vi "CreatePrivateEvents.vi"(8 "error in (no error)":errorcluster, 11 "RemoteControl":refnum<class "RemoteControl.lvclass">) -> (0 "error out":errorcluster, 3 "RemoteControl out":refnum<class "RemoteControl.lvclass">)   [LabVIEW 2016, in "RemoteControl.lvclass"]
doc: "---------------------------------------------------------------\nJKI State Machine Objects™\nhttp://jki.net/state-machine-objects/\nCopyright (C) 2005-2015, JKI <info@jki.net>\nALL RIGHTS RESERVEDJKI State Machine Objects (SMO) 1.0.0.4\nJKI - JKI\nCopyright (c) 2015, JKI"
uses:
  RemoteControl.lvclass
  Typedefs/PrivateEvents--RemoteControl.setAllowedRemoteAddress.ctl
  Typedefs/PrivateEvents--RemoteControl.setAO.ctl
  Typedefs/PrivateEvents--RemoteControl.setAI.ctl
  Typedefs/PrivateEvents--RemoteControl.setResults.ctl
  Typedefs/PrivateEvents--RemoteControl.setTrigger.ctl
  Typedefs/PrivateEvents--RemoteControl.setAOconfig.ctl
  Typedefs/AO-cluster.ctl
  Typedefs/AO_Amp-array.ctl
  Typedefs/AO_DC-array.ctl
  Typedefs/AO_f-array.ctl
  Typedefs/AO_phi-array.ctl
  Typedefs/Function-array.ctl
  Typedefs/Function-enum.ctl
  Typedefs/PrivateEvents--RemoteControl.setREFconfig.ctl
  Typedefs/REF-cluster.ctl
  Typedefs/REF_f-array.ctl
  Typedefs/REF_phi-array.ctl
  Typedefs/PrivateEvents--RemoteControl.setReset.ctl
  Typedefs/PrivateEvents--RemoteControl.setIVmode.ctl
  RemoteControl.lvclass/RemoteControl.ctl
  <vilib>/JKI/JKI SMO/SMO/SMO.lvclass
panel:
  # "For instructions on how to use the JKI State Machine Objects, examples and video tutorials, visit:\nhttp://jki.net/state-machine-objects/\n\nJKI State Machine Objects™\nhttp://jki.net/state-machine-objects/\nCopyright (C) 2005-2015, JKI <info@jki.net>\nALL RIGHTS RESERVED"
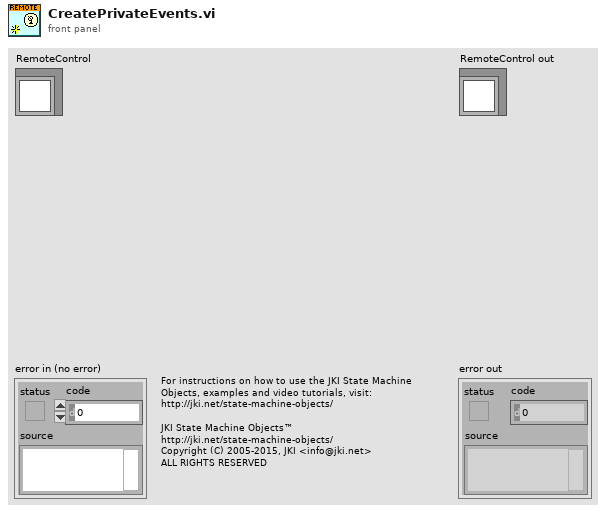
[diagram p1: front panel]
types:
  T1 = typedef "RemoteControl.lvclass/PrivateEvents--RemoteControl.setIVmode.ctl" = bool
  T2 = typedef "RemoteControl.lvclass/PrivateEvents--RemoteControl.setReset.ctl" = bool
  T3 = typedef "RemoteControl.lvclass/PrivateEvents--RemoteControl.setREFconfig.ctl" = cluster{"Channels: Lockin":T4}
  T4 = typedef "REF-cluster.ctl" = cluster{"REF f (Hz)":T5, "REF phi (deg)":T6}
  T5 = typedef "REF_f-array.ctl" = dbl[]
  T6 = typedef "REF_phi-array.ctl" = dbl[]
  T7 = typedef "RemoteControl.lvclass/PrivateEvents--RemoteControl.setAOconfig.ctl" = cluster{"Channels: AO":T8}
  T8 = typedef "AO-cluster.ctl" = cluster{"AO amp (V)":T9, "AO DC (V)":T10, "AO f (Hz)":T11, "AO phi (deg)":T12, "function":T13}
  T9 = typedef "AO_Amp-array.ctl" = dbl[]
  T10 = typedef "AO_DC-array.ctl" = dbl[]
  T11 = typedef "AO_f-array.ctl" = dbl[]
  T12 = typedef "AO_phi-array.ctl" = dbl[]
  T13 = typedef "Function-array.ctl" = T14[]
  T14 = typedef "Function-enum.ctl" = enum16{"Sine Wave", "Triangle Wave", "Square Wave", "Sawtooth Wave"}
  T15 = typedef "RemoteControl.lvclass/PrivateEvents--RemoteControl.setTrigger.ctl" = bool
  T16 = typedef "RemoteControl.lvclass/PrivateEvents--RemoteControl.setResults.ctl" = dbl[][]
  T17 = typedef "RemoteControl.lvclass/PrivateEvents--RemoteControl.setAI.ctl" = waveform(dbl)[]
  T18 = typedef "RemoteControl.lvclass/PrivateEvents--RemoteControl.setAO.ctl" = waveform(dbl)[]
  T19 = typedef "RemoteControl.lvclass/PrivateEvents--RemoteControl.setAllowedRemoteAddress.ctl" = string
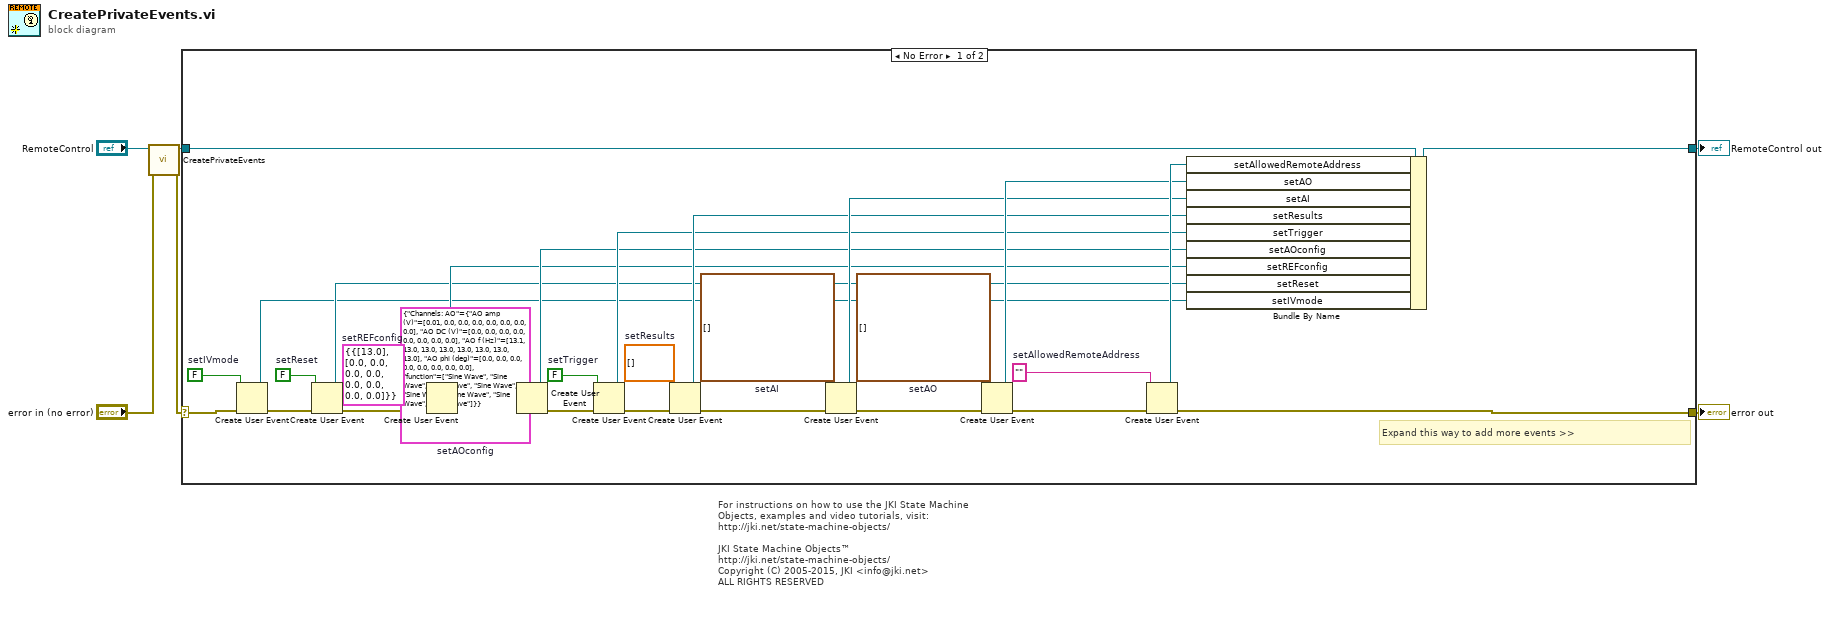
[diagram p0: block diagram]
diagram:
  # "For instructions on how to use the JKI State Machine Objects, examples and video tutorials, visit:\nhttp://jki.net/state-machine-objects/\n\nJKI State Machine Objects™\nhttp://jki.net/state-machine-objects/\nCopyright (C) 2005-2015, JKI <info@jki.net>\nALL RIGHTS RESERVED"
  n1 = call-parent "CreatePrivateEvents.vi"("error in (no error)"="error in (no error)", "SMO"="RemoteControl") -> ("error out"=w1:errorcluster, "SMO out"=w3:refnum<class "RemoteControl.lvclass">)  [unwired: 8 in]
  n2 = case shown="No Error" w1 {
    selector: w1 -> [w35 w38]
    tunnel: [w33 w38] -> w5
    tunnel: [w34 w37] -> w6
    tunnel: w3 -> [w36 w37]
    frame No Error {
      w8 = T1 FALSE  # setIVmode
      w11 = T2 FALSE  # setReset
      w14 = T3 {"Channels: Lockin"={"REF f (Hz)"=[13.0], "REF phi (deg)"=[0.0, 0.0, 0.0, 0.0, 0.0, 0.0, 0.0, 0.0]}}  # setREFconfig
      w17 = T7 {"Channels: AO"={"AO amp (V)"=[0.01, 0.0, 0.0, 0.0, 0.0, 0.0, 0.0, 0.0], "AO DC (V)"=[0.0, 0.0, 0.0, 0.0, 0.0, 0.0, 0.0, 0.0], "AO f (Hz)"=[13.1, 13.0, 13.0, 13.0, 13.0, 13.0, 13.0, 13.0], "AO phi (deg)"=[0.0, 0.0, 0.0, 0.0, 0.0, 0.0, 0.0, 0.0], "function"=[enum."Sine Wave", enum."Sine Wave", enum."Sine Wave", enum."Sine Wave", enum."Sine Wave", enum."Sine Wave", enum."Sine Wave", enum."Sine Wave"]}}  # setAOconfig
      w20 = T15 FALSE  # setTrigger
      w23 = T16 []  # setResults
      w26 = T17 []  # setAI
      w29 = T18 []  # setAO
      w32 = T19 ""  # setAllowedRemoteAddress
      # "Expand this way to add more events >>"
      n3 = Create User Event(user event datatype=w8, error in=w35) -> (user event=w7:refnum<user-event>, error out=w9:errorcluster)
      n4 = Create User Event(user event datatype=w11, error in=w9) -> (user event=w10:refnum<user-event>, error out=w12:errorcluster)
      n5 = Create User Event(user event datatype=w14, error in=w12) -> (user event=w13:refnum<user-event>, error out=w15:errorcluster)
      n6 = Create User Event(user event datatype=w17, error in=w15) -> (user event=w16:refnum<user-event>, error out=w18:errorcluster)
      n7 = Create User Event(user event datatype=w20, error in=w18) -> (user event=w19:refnum<user-event>, error out=w21:errorcluster)
      n8 = Create User Event(user event datatype=w23, error in=w21) -> (user event=w22:refnum<user-event>, error out=w24:errorcluster)
      n9 = Create User Event(user event datatype=w26, error in=w24) -> (user event=w25:refnum<user-event>, error out=w27:errorcluster)
      n10 = Create User Event(user event datatype=w29, error in=w27) -> (user event=w28:refnum<user-event>, error out=w30:errorcluster)
      n11 = Create User Event(user event datatype=w32, error in=w30) -> (user event=w31:refnum<user-event>, error out=w33:errorcluster)
      n12 = Bundle By Name(cluster=w36, "setAllowedRemoteAddress"=w31, "setAO"=w28, "setAI"=w25, "setResults"=w22, "setTrigger"=w19, "setAOconfig"=w16, "setREFconfig"=w13, "setReset"=w10, "setIVmode"=w7) -> (w34:refnum<class "RemoteControl.lvclass">)
    }
    frame Error {
    }
  }
  "error out" <- w5
  "RemoteControl out" <- w6
